vi "COM.vi"(8 "error in (no error)":errorcluster, 10 "Command":string, 11 "VISA Refnum in":refnum<visa-resource-name>="COM3") -> (0 "error out":errorcluster, 2 "Response":string="\r\n", 3 "VISA Refnum out":refnum<visa-resource-name>)   [LabVIEW 2019, in "KH7008.lvlib"]
uses:
  KH7008.lvlib
panel:
  out "read buffer":string
  out "Retries":i32
  out "return count":u32
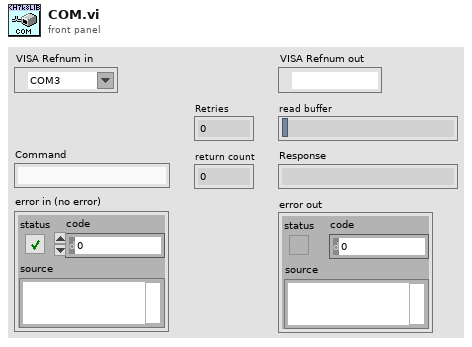
[diagram p1: front panel]
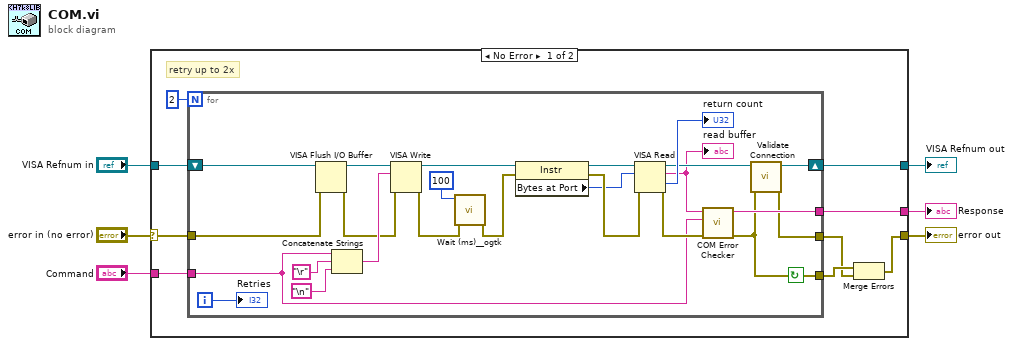
[diagram p0: block diagram]
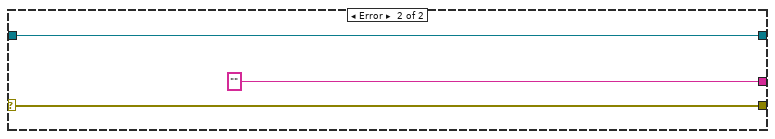
[diagram p2: hidden frame]
diagram:
  n1 = case shown="No Error" "error in (no error)" {
    selector: "error in (no error)" -> [w11 w40]
    tunnel: "VISA Refnum in" -> [w12 w41]
    tunnel: "Command" -> [w13 _]
    tunnel: [w9 w40] -> w4
    tunnel: [w15 "" ("String")] -> w3
    tunnel: [w14 w41] -> w2
    frame No Error {
      # "retry up to 2x"
      n2 = for {
        N: 2 -> [_]
        tunnel: w11 -> [w23]
        shift-right: [w21] -> w14
        shift-left: w12 -> [w32]
        tunnel: [w20] -> w7
        tunnel: w13 -> [w16]
        tunnel: [w38] -> w15
        tunnel: [w17] -> w8
        i -> [w19]
        stop <- w17 continue-if-true
        n3 = VISA Flush I/O Buffer(VISA resource name=w32, error in (no error)=w23) -> (VISA resource name out=w33:refnum<visa-resource-name>, error out=w34:errorcluster)  [unwired: 1 in]
        n4 = Concatenate Strings(w16, "\r", "\n") -> (w37:string)
        n5 = VISA Write(VISA resource name=w33, write buffer=w37, error in (no error)=w34) -> (VISA resource name out=w29:refnum<visa-resource-name>, error out=w30:errorcluster)  [unwired: 1 out]
        n6 = call <userlib>:"Wait (ms)__ogtk.vi"("error in (no error)"=w30, "milliseconds to wait"=u32 100) -> ("error out"=w27:errorcluster)  [unwired: 8 in, 1 out]
        n7 = property class="Instr"(reference=w29, error in=w27) -> (reference out=w28:refnum<visa-resource-name>, error out=w26:errorcluster, "Bytes at Port"=w24:u32)
        n8 = VISA Read(VISA resource name=w28, byte count=w24, error in (no error)=w26) -> (VISA resource name out=w22:refnum<visa-resource-name>, read buffer=w18:string, return count=→"return count":u32, error out=w39:errorcluster)
        "read buffer" <- w18
        n9 = call "COM Error Checker.vi"("error in (no error)"=w39, "Command"=w16, "Response"=w18) -> ("error out"=w17:errorcluster, "Response"=w38:string)  [unwired: 7 in]
        n10 = call "Validate Connection.vi"("error in (no error)"=w17, "VISA Refnum in"=w22) -> ("error out"=w20:errorcluster, "VISA Refnum out"=w21:refnum<visa-resource-name>)  [unwired: 8 in]
        "Retries" <- w19
      }
      n11 = Merge Errors(w8, w7) -> (w9:errorcluster)
    }
    frame Error {
    }
  }
  "error out" <- w4
  "Response" <- w3
  "VISA Refnum out" <- w2
